vi "Serialize - JSON.vi"(8 "error in":errorcluster, 11 "mTEC Data in":refnum<class "mTEC Data.lvclass">) -> (0 "error out":errorcluster, 2 "Serialized JSON":string, 3 "mTEC Data out":refnum<class "mTEC Data.lvclass">)   [LabVIEW 2014, in "Meerstetter Lib.lvlib" / "mTEC Data.lvclass"]
uses:
  mTEC Data.lvclass
  mTEC Data.lvclass/mTEC Data.ctl
  Read Tobj.vi
  Read Tsink.vi
  Read Vout.vi
  reusable/Data/Data.lvlibp/Read Data ID.vi
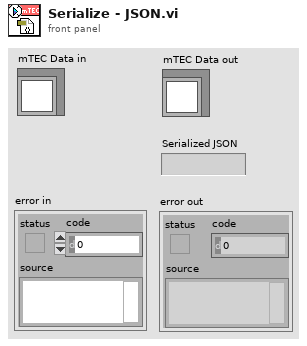
[diagram p1: front panel]
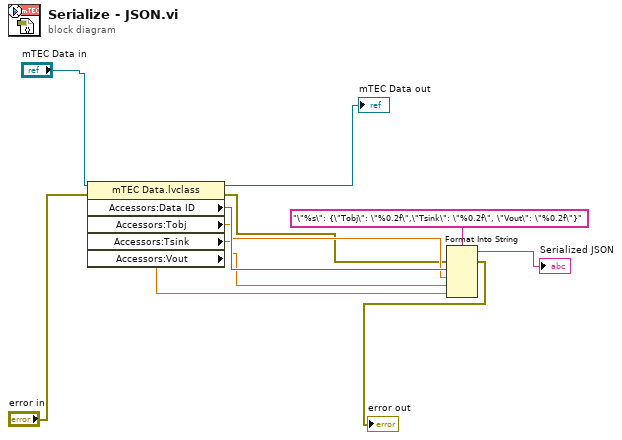
[diagram p0: block diagram]
diagram:
  n1 = property class="mTEC Data.lvclass"(reference="mTEC Data in", error in="error in") -> (reference out=→"mTEC Data out":refnum<class "mTEC Data.lvclass">, error out=w2:errorcluster, "Accessors:Data ID"=w6:string, "Accessors:Tobj"=w5:dbl, "Accessors:Tsink"=w4:dbl, "Accessors:Vout"=w3:dbl)
  n2 = Format Into String(format string="\"%s\": {\"Tobj\": \"%0.2f\",\"Tsink\": \"%0.2f\", \"Vout\": \"%0.2f\"}", error in=w2, w6, w5, w4, w3) -> (resulting string=→"Serialized JSON":string, error out=→"error out":errorcluster)  [unwired: 1 in]
